vi "Init.vi"(9 "Queue":refnum<class "Queue.lvclass">, 10 "Self Queue Alias":string) -> (3 "Create Queue Msg Strategy out":refnum<class "Create Queue Msg Strategy.lvclass">)   [LabVIEW 2021, in "jettl Msg Create Queue.lvlib" / "Create Queue Msg Strategy.lvclass"]
uses:
  Create Queue Msg Strategy.lvclass
  jettl/Queue/Queue.lvclass
  Create Queue Msg Strategy.lvclass/Create Queue Msg Strategy.ctl
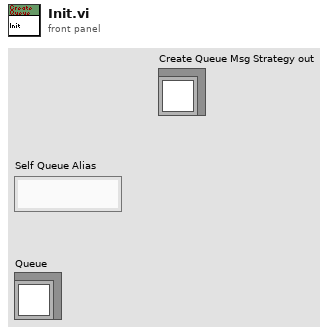
[diagram p1: front panel]
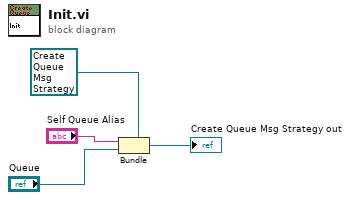
[diagram p0: block diagram]
diagram:
  n1 = Bundle(cluster=refnum<class "Create Queue Msg Strategy.lvclass"> refnum ("Create Msg in"), "Self Queue Alias", "Queue") -> (→"Create Queue Msg Strategy out":refnum<class "Create Queue Msg Strategy.lvclass">)
